vi "Extract Data.vi"(10 "index in":i32, 11 "Array In":string[](array[string])) -> (2 "Data":string, 3 "Array Out":string[](array[string]))   [LabVIEW 2013, in "Mercury iXX.lvlib" / "Level Meter.lvlib"]
uses:
  <instrlib>/Mercury iXX/Public/Libraries/Level Meter.lvlib
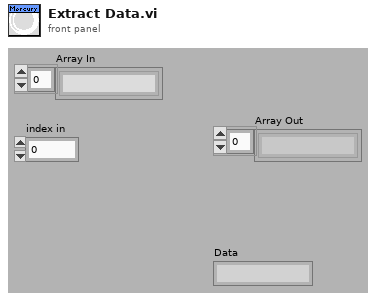
[diagram p1: front panel]
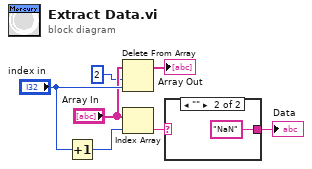
[diagram p0: block diagram]
diagram:
  n1 = Increment(x="index in") -> (x+1=w3:i32)
  n2 = Delete From Array(array="Array In", length=2, index="index in") -> (array with subset deleted=→"Array Out":string[])  [unwired: 1 out]
  n3 = Index Array(array="Array In", index=w3) -> (element=w2:string)
  n4 = case shown="\"\"" w2 {
    selector: w2 -> [w8 _]
    tunnel: [w8 "NaN"] -> w1
    frame Default {
    }
    frame "" {
    }
  }
  "Data" <- w1
